vi "Unpack list of strings.vi"(8 "error in (no error)":errorcluster, 11 "Python Toolkit in":refnum<class "Python Toolkit.lvclass">) -> (0 "error out":errorcluster, 2 "cards":string[](array[string]), 3 "Python Toolkit out":refnum<class "Python Toolkit.lvclass">)   [LabVIEW 2018, in "Python Toolkit.lvclass"]
doc: "Get the value returned by a python function\n\nThis value is structured as a array of strings"
uses:
  Python Toolkit.lvclass
  Python Toolkit.lvclass/Python Toolkit.ctl
  <vilib>/Enthought/Python Integration Toolkit/api/Unpack String Array.vi
  <vilib>/Enthought/Python Integration Toolkit/Python Integration Toolkit.lvlib
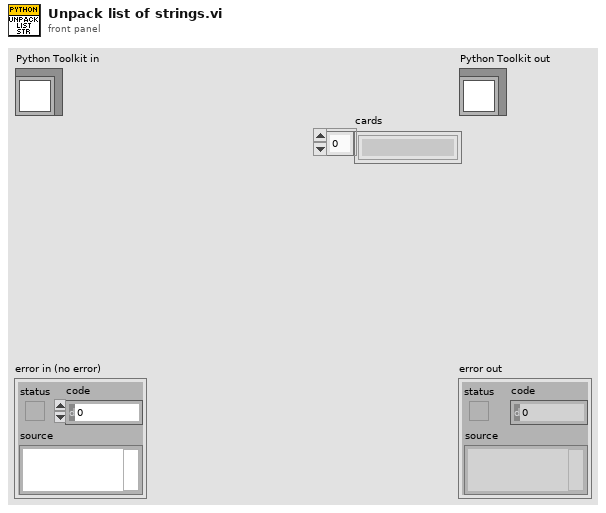
[diagram p1: front panel]
types:
  T1 = typedef "Python Integration Toolkit.lvlib/Session ID.ctl" = u64
  T2 = typedef "Python Integration Toolkit.lvlib/Python Objects.ctl" = variant
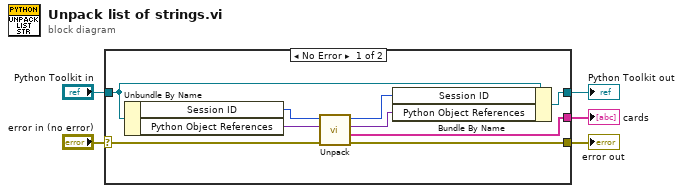
[diagram p0: block diagram]
diagram:
  n1 = case shown="No Error" "error in (no error)" {
    selector: "error in (no error)" -> [w14 w16]
    tunnel: [w13 w16] -> w4
    tunnel: [w8 w15] -> w2
    tunnel: "Python Toolkit in" -> [w9 w15]
    tunnel: [w10 _] -> w1
    frame No Error {
      n2 = Unbundle By Name(w9) -> ("Session ID"=w12:T1, "Python Object References"=w11:T2)
      n3 = call-poly <vilib>:"Unpack.vi"("error in (no error)"=w14, "Python Object References In"=w11, "Session ID"=w12) -> ("error out"=w13:errorcluster, "Value"=w10:string[], "Python Object References Out"=w7:T2, "Session ID out"=w6:T1)  [unwired: 5 in]
      n4 = Bundle By Name(cluster=w9, "Session ID"=w6, "Python Object References"=w7) -> (w8:refnum<class "Python Toolkit.lvclass">)
    }
    frame Error {
    }
  }
  "error out" <- w4
  "Python Toolkit out" <- w2
  "cards" <- w1
